vi "Test Retriggerable.vi"() -> ()   [LabVIEW 2014]
uses:
  <vilib>/DAQmx/configure/timing.llb/DAQmx Timing (Implicit).vi
  <vilib>/DAQmx/configure/timing.llb/DAQmx Timing (Sample Clock).vi
  <vilib>/DAQmx/read.llb/DAQmx Read (Analog 2D DBL NChan NSamp).vi
  <resource>/objmgr/daqmx.rc
panel:
  out "error out 6":errorcluster
  out "error out 5":errorcluster
  out "size(s) 2":i32[](array[numeric])
  out "size(s)":i32[](array[numeric])
  out "error out 4":errorcluster
  out "error out 3":errorcluster
  out "error out 2":errorcluster
  out "error out":errorcluster
  in  "Stop Button":bool
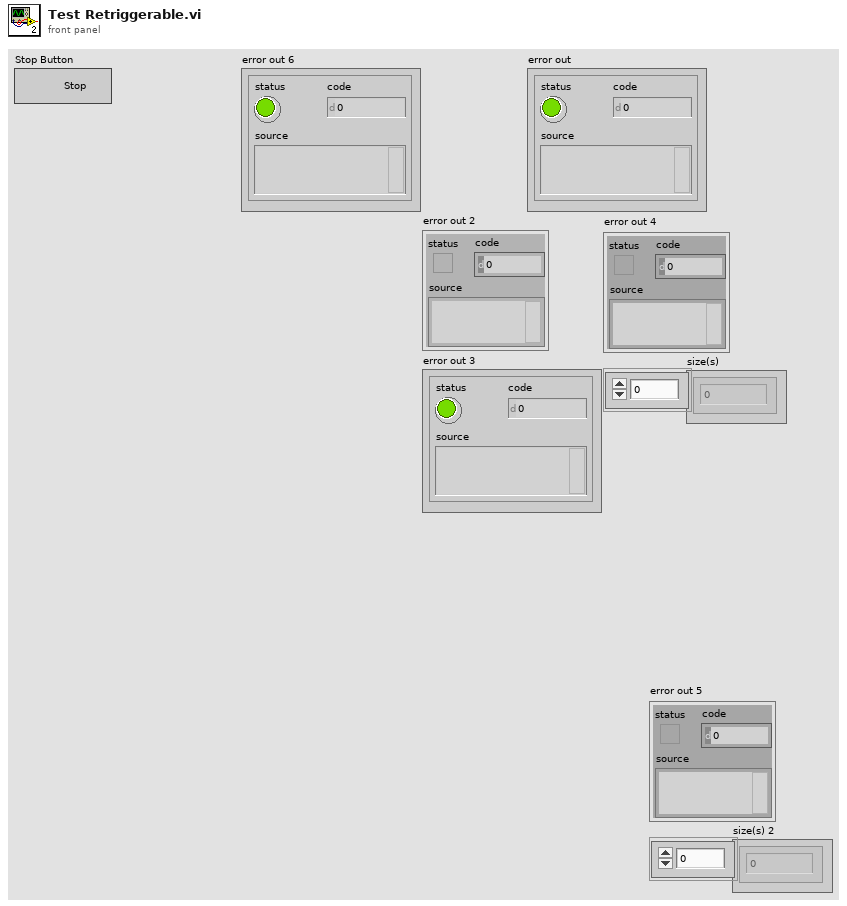
[diagram p1: front panel]
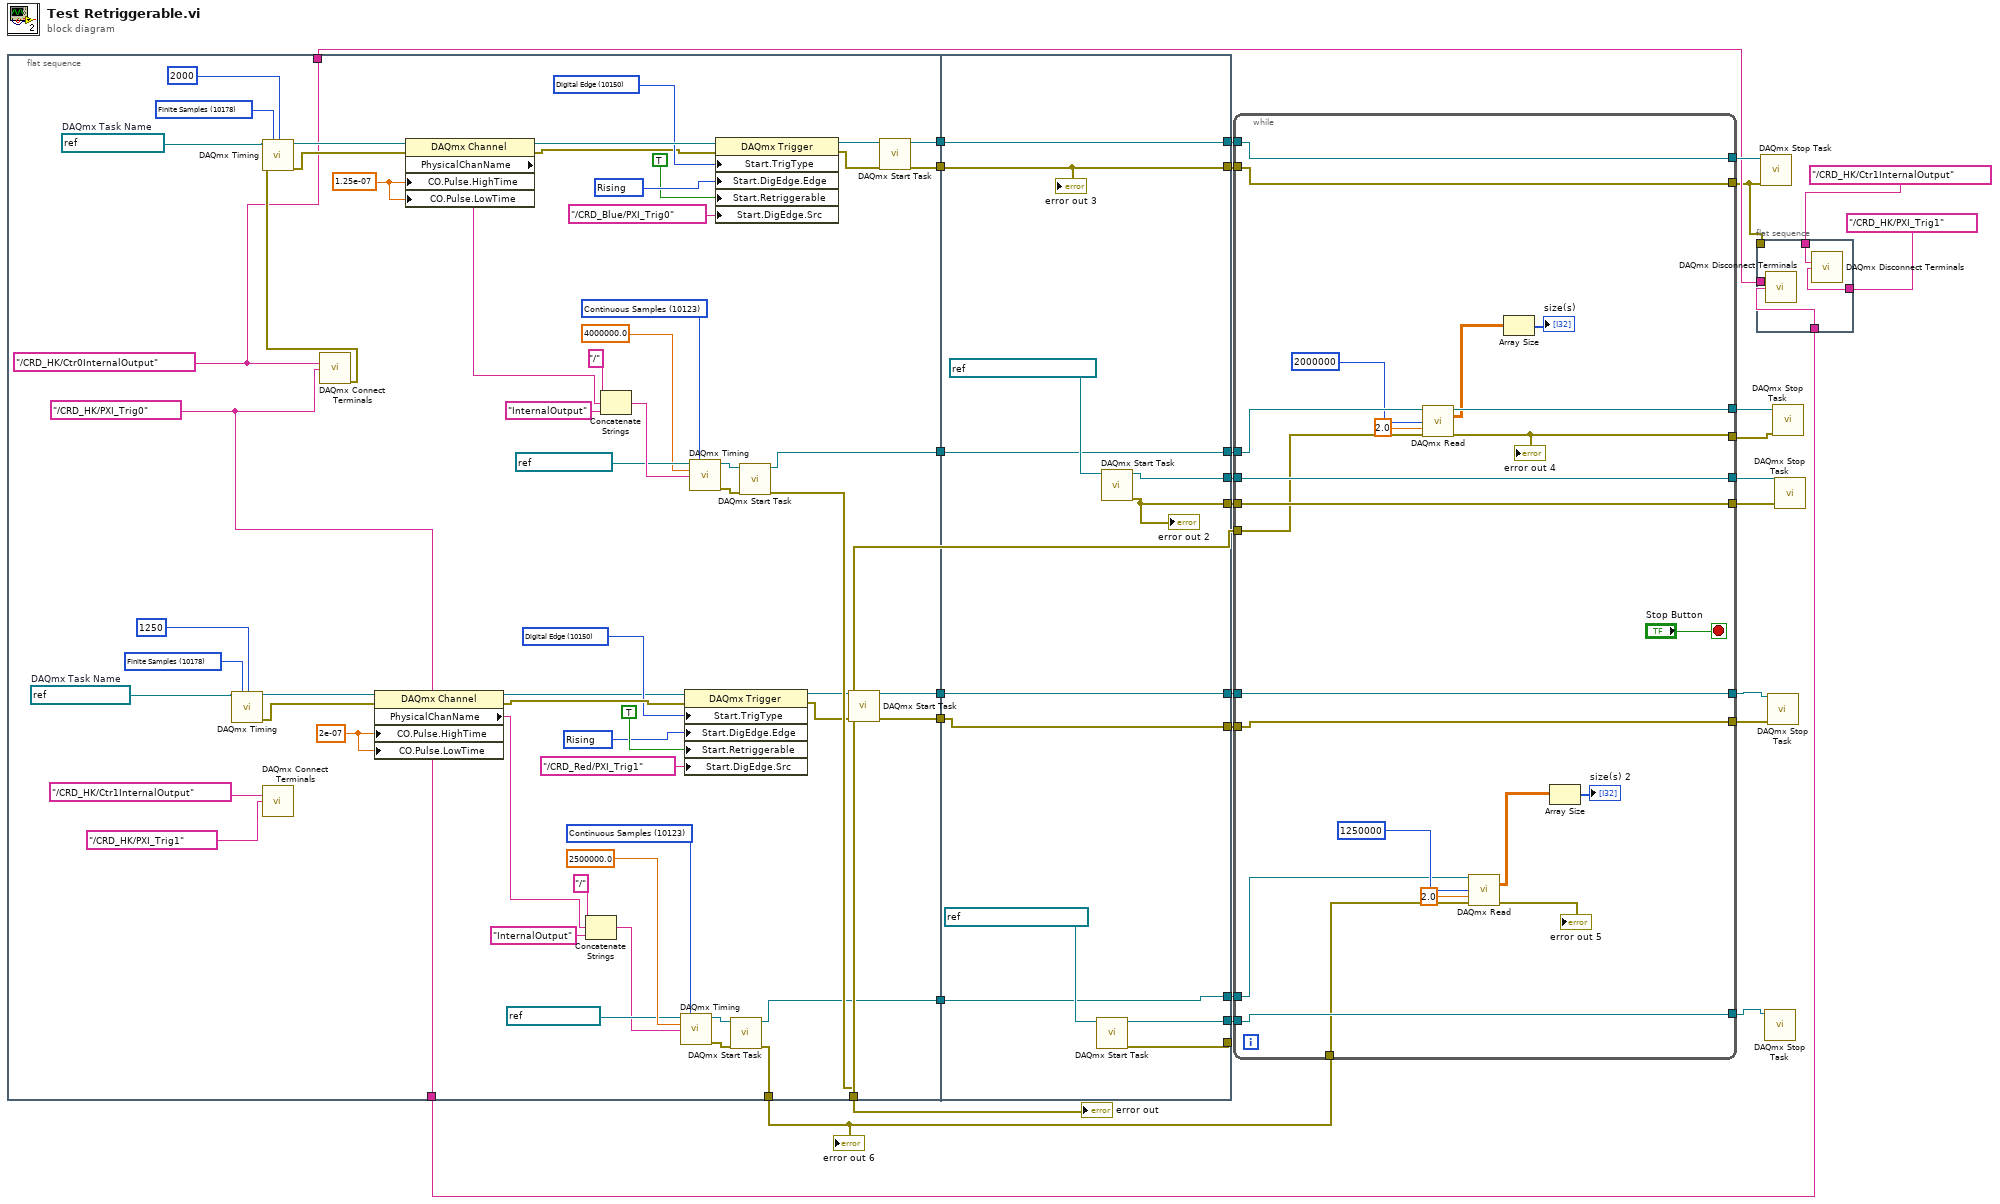
[diagram p0: block diagram]
diagram:
  n1 = flat-sequence {
    tunnel: [w70] -> w28
    tunnel: [w69] -> w27
    tunnel: [w66] -> w26
    tunnel: [w65] -> w17
    tunnel: [w62] -> w16
    tunnel: [w61] -> w15
    tunnel: [w35] -> w13
    tunnel: [w33] -> w9
    tunnel: [w32] -> w8
    tunnel: [w31] -> w5
    tunnel: [w100] -> w29
    tunnel: [w101] -> w30
    tunnel: w28 -> [w101]
    tunnel: w27 -> [w100]
    tunnel: w26 -> [w98]
    tunnel: [w98] -> w25
    tunnel: [w97] -> w24
    tunnel: [w96] -> w23
    tunnel: w13 -> [w94]
    tunnel: [w94] -> w10
    tunnel: [w93] -> w12
    tunnel: w8 -> [w92]
    tunnel: [w92] -> w7
    tunnel: w5 -> [w91]
    tunnel: [w91] -> w4
    tunnel: [w90] -> _
    frame #0 {
      w43 = 10123 items=["Finite Samples"=10178, "Continuous Samples"=10123, "Hardware Timed Single Point"=12522] ("sample mode")
      w53 = 10280 items=["Rising"=10280, "Falling"=10171] ("Ref.DigEdge.Edge")
      w52 = 10150 items=["Analog Edge"=10099, "Digital Edge"=10150, "Digital Pattern"=10398, "Analog Window"=10103, "None"=10230] ("Ref.TrigType")
      w50 = 2e-07 ("CO.Pulse.HighTime")
      w47 = 10178 items=["Finite Samples"=10178, "Continuous Samples"=10123, "Hardware Timed Single Point"=12522] ("sample mode")
      w46 = refnum<k21> "CRDS Red Clk"  # DAQmx Task Name
      w60 = 10123 items=["Finite Samples"=10178, "Continuous Samples"=10123, "Hardware Timed Single Point"=12522] ("sample mode")
      w61 = tag "/CRD_HK/PXI_Trig0" ("destination terminal")
      w62 = tag "/CRD_HK/Ctr0InternalOutput" ("source terminal")
      w76 = 10280 items=["Rising"=10280, "Falling"=10171] ("Ref.DigEdge.Edge")
      w77 = 10150 items=["Analog Edge"=10099, "Digital Edge"=10150, "Digital Pattern"=10398, "Analog Window"=10103, "None"=10230] ("Ref.TrigType")
      w85 = 1.25e-07 ("CO.Pulse.HighTime")
      w88 = 10178 items=["Finite Samples"=10178, "Continuous Samples"=10123, "Hardware Timed Single Point"=12522] ("sample mode")
      w89 = refnum<k21> "CRDS Blue Clk"  # DAQmx Task Name
      n2 = call-poly <vilib>:"DAQmx Timing.vi"("task/channels in"=w46, "sample mode"=w47, "samples per channel"=1250) -> ("task out"=w49:refnum<k21>, "error out"=w55:errorcluster)  [unwired: 11 in]
      n3 = call <vilib>:"DAQmx Connect Terminals.vi"("source terminal"=tag "/CRD_HK/Ctr1InternalOutput", "destination terminal"=tag "/CRD_HK/PXI_Trig1") -> ()  [unwired: 13 in, 1 out]
      n4 = call <vilib>:"DAQmx Connect Terminals.vi"("source terminal"=w62, "destination terminal"=w61) -> ("error out"=w63:errorcluster)  [unwired: 13 in]
      n5 = call-poly <vilib>:"DAQmx Timing.vi"("task/channels in"=w89, "sample mode"=w88, "samples per channel"=2000, "error in"=w63) -> ("task out"=w86:refnum<k21>, "error out"=w74:errorcluster)  [unwired: 10 in]
      n6 = property class="DAQmx Channel"(reference=w49, error in=w55, "CO.Pulse.HighTime"=w50, "CO.Pulse.LowTime"=w50) -> (reference out=w51:refnum<k21>, error out=w56:errorcluster, "PhysicalChanName"=w34:tag)
      n7 = property class="DAQmx Channel"(reference=w86, error in=w74, "CO.Pulse.HighTime"=w85, "CO.Pulse.LowTime"=w85) -> (reference out=w78:refnum<k21>, error out=w73:errorcluster, "PhysicalChanName"=w82:tag)
      n8 = Concatenate Strings("/" ("string"), w34, "InternalOutput" ("string")) -> (w38:string)
      n9 = Concatenate Strings("/" ("string"), w82, "InternalOutput" ("string")) -> (w81:string)
      n10 = call-poly <vilib>:"DAQmx Timing.vi"("task/channels in"=refnum<k21> "CRDS Red AI", "sample mode"=w43, "rate"=2500000.0, "source"=w38) -> ("task out"=w41:refnum<k21>, "error out"=w42:errorcluster)  [unwired: 10 in]
      n11 = property class="DAQmx Trigger"(reference=w51, error in=w56, "Start.TrigType"=w52, "Start.DigEdge.Edge"=w53, "Start.Retriggerable"=TRUE, "Start.DigEdge.Src"=tag "/CRD_Red/PXI_Trig1") -> (reference out=w57:refnum<k21>, error out=w58:errorcluster)
      n12 = call-poly <vilib>:"DAQmx Timing.vi"("task/channels in"=refnum<k21> "CRDS Blue AI", "sample mode"=w60, "rate"=4000000.0, "source"=w81) -> ("task out"=w68:refnum<k21>, "error out"=w67:errorcluster)  [unwired: 10 in]
      n13 = property class="DAQmx Trigger"(reference=w78, error in=w73, "Start.TrigType"=w77, "Start.DigEdge.Edge"=w76, "Start.Retriggerable"=TRUE, "Start.DigEdge.Src"=tag "/CRD_Blue/PXI_Trig0") -> (reference out=w72:refnum<k21>, error out=w71:errorcluster)
      n14 = call <vilib>:"DAQmx Start Task.vi"("task/channels in"=w41, "error in"=w42) -> ("task out"=w35:refnum<k21>, "error out"=w33:errorcluster)  [unwired: 12 in]
      n15 = call <vilib>:"DAQmx Start Task.vi"("task/channels in"=w68, "error in"=w67) -> ("task out"=w66:refnum<k21>, "error out"=w65:errorcluster)  [unwired: 12 in]
      n16 = call <vilib>:"DAQmx Start Task.vi"("task/channels in"=w57, "error in"=w58) -> ("task out"=w32:refnum<k21>, "error out"=w31:errorcluster)  [unwired: 12 in]
      n17 = call <vilib>:"DAQmx Start Task.vi"("task/channels in"=w72, "error in"=w71) -> ("task out"=w70:refnum<k21>, "error out"=w69:errorcluster)  [unwired: 12 in]
    }
    frame #1 {
      n18 = call <vilib>:"DAQmx Start Task.vi"("task/channels in"=refnum<k21> "CRD Red Laser Output") -> ("task out"=w93:refnum<k21>, "error out"=w90:errorcluster)  [unwired: 13 in]
      n19 = call <vilib>:"DAQmx Start Task.vi"("task/channels in"=refnum<k21> "CRD Blue Laser Output") -> ("task out"=w97:refnum<k21>, "error out"=w96:errorcluster)  [unwired: 13 in]
      "error out 2" <- w96
      "error out 3" <- w100
    }
  }
  n20 = while {
    tunnel: w30 -> [w116]
    tunnel: w29 -> [w115]
    tunnel: w25 -> [w121]
    tunnel: w24 -> [w123]
    tunnel: w23 -> [w122]
    tunnel: [w123] -> w22
    tunnel: [w122] -> w21
    tunnel: [w119] -> w20
    tunnel: [w118] -> w19
    tunnel: [w116] -> w18
    tunnel: [w115] -> w14
    tunnel: w17 -> [w114]
    tunnel: w12 -> [w111]
    tunnel: [w111] -> w11
    tunnel: w10 -> [w105]
    tunnel: w9 -> [w104]
    tunnel: w7 -> [w103]
    tunnel: [w103] -> w6
    tunnel: w4 -> [w102]
    tunnel: [w102] -> w3
    stop <- "Stop Button" stop-if-true
    n21 = call-poly <vilib>:"DAQmx Read.vi"("task/channels in"=w121, "number of samples per channel"=2000000, "timeout"=2.0, "error in"=w114) -> ("task out"=w119:refnum<k21>, "data"=w113:dbl[][], "error out"=w118:errorcluster)  [unwired: 9 in]
    "error out 4" <- w118
    n22 = call-poly <vilib>:"DAQmx Read.vi"("task/channels in"=w105, "number of samples per channel"=1250000, "timeout"=2.0, "error in"=w104) -> ("data"=w109:dbl[][], "error out"=→"error out 5":errorcluster)  [unwired: 9 in, 1 out]
    n23 = Array Size(array=w113) -> (size(s)=→"size(s)":i32[])
    n24 = Array Size(array=w109) -> (size(s)=→"size(s) 2":i32[])
  }
  n25 = flat-sequence {
    tunnel: w16 -> [w128]
    tunnel: w15 -> [w127]
    tunnel: w14 -> [_]
    tunnel: tag "/CRD_HK/Ctr1InternalOutput" ("source terminal") -> [w126]
    tunnel: tag "/CRD_HK/PXI_Trig1" ("destination terminal") -> [w125]
    frame #0 {
      n26 = call <vilib>:"DAQmx Disconnect Terminals.vi"("source terminal"=w128, "destination terminal"=w127) -> ()  [unwired: 13 in, 1 out]
      n27 = call <vilib>:"DAQmx Disconnect Terminals.vi"("source terminal"=w126, "destination terminal"=w125) -> ()  [unwired: 13 in, 1 out]
    }
  }
  n28 = call <vilib>:"DAQmx Stop Task.vi"("task/channels in"=w18, "error in"=w14) -> ()  [unwired: 12 in, 2 out]
  n29 = call <vilib>:"DAQmx Stop Task.vi"("task/channels in"=w11) -> ()  [unwired: 13 in, 2 out]
  n30 = call <vilib>:"DAQmx Stop Task.vi"("task/channels in"=w6, "error in"=w3) -> ()  [unwired: 12 in, 2 out]
  n31 = call <vilib>:"DAQmx Stop Task.vi"("task/channels in"=w20, "error in"=w19) -> ()  [unwired: 12 in, 2 out]
  n32 = call <vilib>:"DAQmx Stop Task.vi"("task/channels in"=w22, "error in"=w21) -> ()  [unwired: 12 in, 2 out]
  "error out" <- w17
  "error out 6" <- w9
